vi "Read Rectangle.vi"(0 "GetPageSizeWithRotation":refnum<k24>, 7 "Pages dimensions [ ] IN":T1[](array[typedef]) {"Page Size" items=["Custom", "LETTER", "NOTE", "LEGAL", "TABLOID", "EXECUTIVE", "POSTCARD", "A0", "A1", "A2", "A3", "A4", "A5", "A6", "A7", "A8", "A9", "A10", "B0", "B1", "B2", "B3", "B4", "B5", "B6", "B7", "B8", "B9", "B10", "ARCH_E", "ARCH_D", "ARCH_C", "ARCH_B", "ARCH_A", "FLSA", "FLSE", "HALFLETTER", "_11X17", "ID_1", "ID_2", "ID_3", "LEDGER", "CROWN_QUARTO", "LARGE_CROWN_QUARTO", "DEMY_QUARTO", "ROYAL_QUARTO", "CROWN_OCTAVO", "LARGE_CROWN_OCTAVO", "DEMY_OCTAVO", "ROYAL_OCTAVO", "SMALL_PAPERBACK", "PENGUIN_SMALL_PAPERBACK", "PENGUIN_LARGE_PAPERBACK"]}, 11 "error in (no error)":errorcluster, 13 "Start at page":i32=1) -> (8 "Pages dimensions [ ] OUT":T1[](array[typedef]) {"Page Size" items=["Custom", "LETTER", "NOTE", "LEGAL", "TABLOID", "EXECUTIVE", "POSTCARD", "A0", "A1", "A2", "A3", "A4", "A5", "A6", "A7", "A8", "A9", "A10", "B0", "B1", "B2", "B3", "B4", "B5", "B6", "B7", "B8", "B9", "B10", "ARCH_E", "ARCH_D", "ARCH_C", "ARCH_B", "ARCH_A", "FLSA", "FLSE", "HALFLETTER", "_11X17", "ID_1", "ID_2", "ID_3", "LEDGER", "CROWN_QUARTO", "LARGE_CROWN_QUARTO", "DEMY_QUARTO", "ROYAL_QUARTO", "CROWN_OCTAVO", "LARGE_CROWN_OCTAVO", "DEMY_OCTAVO", "ROYAL_OCTAVO", "SMALL_PAPERBACK", "PENGUIN_SMALL_PAPERBACK", "PENGUIN_LARGE_PAPERBACK"]}, 15 "error out":errorcluster)   [LabVIEW 2019]
doc: "Developed by Jean-Marc Simard\nCopyright © 2012, Exaprom Inc.\nAll rights reserved.\nLicense: BSD\n\nWith iTextSharp 4.1.6 (http://itextsharp.sourceforge.net)\nunder Mozilla Public License Version 1.1\n(http://www.mozilla.org/MPL/MPL-1.1.html)"
uses:
  C:/Program Files/National Instruments/LabVIEW 2019/user.lib/Exaprom PDF/DLL/itextsharp.dll
  DLL/itextsharp.dll
  <userlib>/Exaprom PDF/Controls/Page Controls/Page dimensions.ctl
  <userlib>/Exaprom PDF/Controls/Page Controls/Page size.ctl
  <userlib>/Exaprom PDF/Controls/Page Controls/Page Orientation.ctl
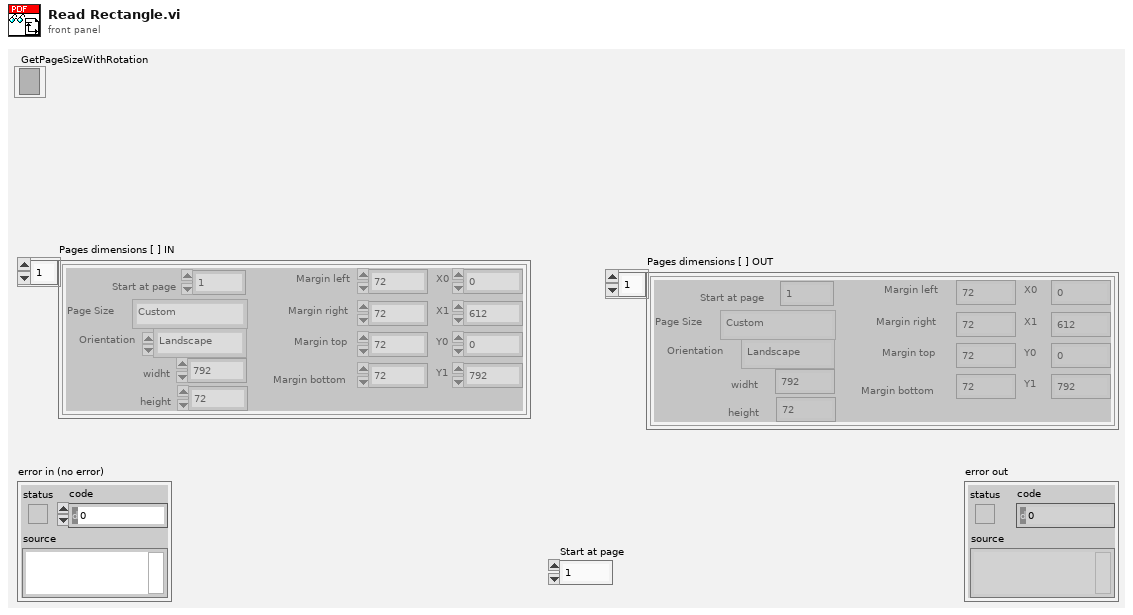
[diagram p1: front panel]
types:
  T1 = typedef "Page dimensions.ctl" = cluster{"Start at page":i32, "Page Size":T2, "Orientation":T3, "widht":sgl, "height":sgl, "Margin left":sgl, "Margin right":sgl, "Margin top":sgl, "Margin bottom":sgl, "X0":sgl, "X1":sgl, "Y0":sgl, "Y1":sgl}
  T2 = typedef "Page size.ctl" = i32
  T3 = typedef "Page Orientation.ctl" = enum16{"Portrait", "Landscape"}
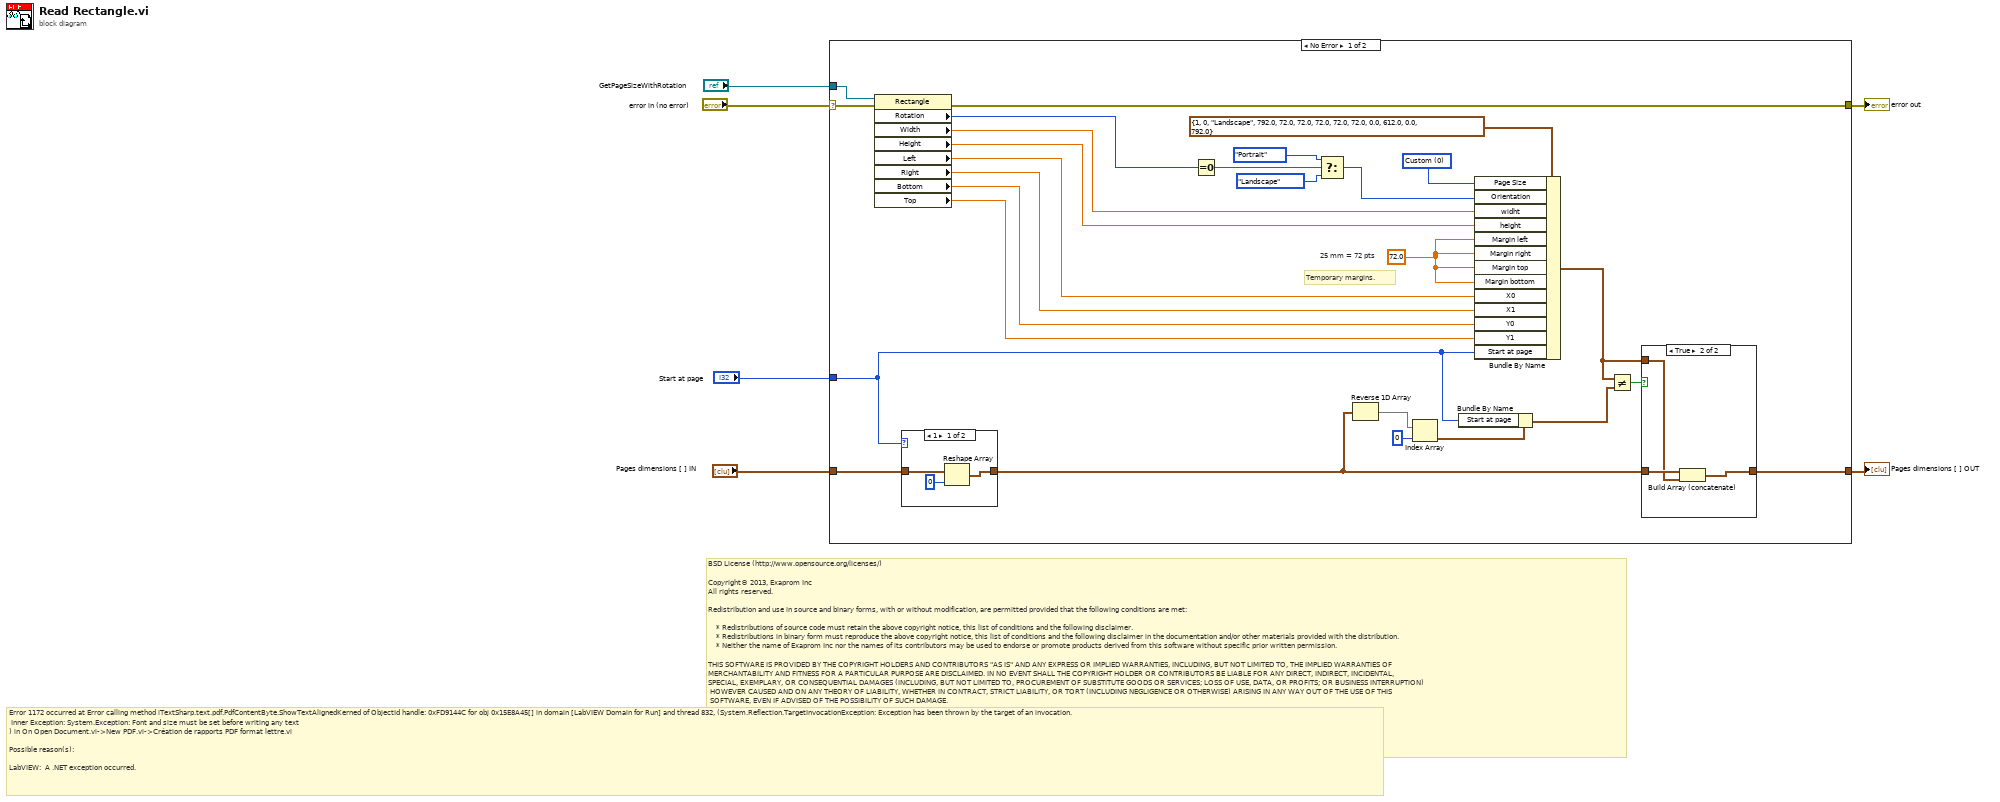
[diagram p0: block diagram]
diagram:
  # "Error 1172 occurred at Error calling method iTextSharp.text.pdf.PdfContentByte.ShowTextAlignedKerned of ObjectId handle: 0xFD9144C for obj 0x15E8A45[] in domain [LabVIEW Domain for Run] and thread 832, (System.Reflection.TargetInvocationException: Exception has been thrown by the target of an invocation.\n\tInner Exception: System.Exception: Font and size must be set before writing any text\n) in On Open Document.vi->New PDF.vi->Création de rapports PDF format lettre.vi\n\nPossible reason(s):\n\nLabVIEW:  A .NET exception occurred."
  # "BSD License (http://www.opensource.org/licenses/)\n\nCopyright© 2013, Exaprom Inc\nAll rights reserved.\n\nRedistribution and use in source and binary forms, with or without modification, are permitted provided that the following conditions are met:\n\n    * Redistributions of source code must retain the above copyright notice, this list of conditions and the following disclaimer.\n    * Redistributions in binary form must reproduce the above copyright notice, this list of conditions and the following disclaimer in the documentation and/or other materials provided with the distribution.\n    * Neither the name of Exaprom Inc nor the names of its contributors may be used to endorse or promote products derived from this software without specific prior written permission.\n\nTHIS SOFTWARE IS PROVIDED BY THE COPYRIGHT HOLDERS AND CONTRIBUTORS \"AS IS\" AND ANY EXPRESS OR IMPLIED WARRANTIES, INCLUDING, BUT NOT LIMITED TO, THE IMPLIED WARRANTIES OF \nMERCHANTABILITY AND FITNESS FOR A PARTICULAR PURPOSE ARE DISCLAIMED. IN NO EVENT SHALL THE COPYRIGHT HOLDER OR CONTRIBUTORS BE LIABLE FOR ANY DIRECT, INDIRECT, INCIDENTAL,\nSPECIAL, EXEMPLARY, OR CONSEQUENTIAL DAMAGES (INCLUDING, BUT NOT LIMITED TO, PROCUREMENT OF SUBSTITUTE GOODS OR SERVICES; LOSS OF USE, DATA, OR PROFITS; OR BUSINESS INTERRUPTION)\n HOWEVER CAUSED AND ON ANY THEORY OF LIABILITY, WHETHER IN CONTRACT, STRICT LIABILITY, OR TORT (INCLUDING NEGLIGENCE OR OTHERWISE) ARISING IN ANY WAY OUT OF THE USE OF THIS\n SOFTWARE, EVEN IF ADVISED OF THE POSSIBILITY OF SUCH DAMAGE."
  n1 = case shown="No Error" "error in (no error)" {
    selector: "error in (no error)" -> [w33 w42]
    tunnel: [w26 w42] -> w6
    tunnel: "GetPageSizeWithRotation" -> [w32 _]
    tunnel: "Start at page" -> [w7 _]
    tunnel: "Pages dimensions [ ] IN" -> [w10 _]
    tunnel: [w11 _] -> w1
    frame No Error {
      w21 = sgl 72.0  # 25 mm = 72 pts
      w24 = T2 0 items=["Custom", "LETTER", "NOTE", "LEGAL", "TABLOID", "EXECUTIVE", "POSTCARD", "A0", "A1", "A2", "A3", "A4", "A5", "A6", "A7", "A8", "A9", "A10", "B0", "B1", "B2", "B3", "B4", "B5", "B6", "B7", "B8", "B9", "B10", "ARCH_E", "ARCH_D", "ARCH_C", "ARCH_B", "ARCH_A", "FLSA", "FLSE", "HALFLETTER", "_11X17", "ID_1", "ID_2", "ID_3", "LEDGER", "CROWN_QUARTO", "LARGE_CROWN_QUARTO", "DEMY_QUARTO", "ROYAL_QUARTO", "CROWN_OCTAVO", "LARGE_CROWN_OCTAVO", "DEMY_OCTAVO", "ROYAL_OCTAVO", "SMALL_PAPERBACK", "PENGUIN_SMALL_PAPERBACK", "PENGUIN_LARGE_PAPERBACK"] ("Page Size")
      # "Temporary margins."
      n2 = property class="Rectangle"(reference=w32, error in=w33) -> (error out=w26:errorcluster, "Rotation"=w31:i32, "Width"=w23:sgl, "Height"=w22:sgl, "Left"=w20:sgl, "Right"=w19:sgl, "Bottom"=w18:sgl, "Top"=w17:sgl)  [unwired: 1 out]
      n3 = case shown="1" w7 {
        tunnel: w10 -> [w36 w37]
        tunnel: [w35 w37] -> w8
        frame 1 {
          n4 = Reshape Array(w36, 0 ("dimension size")) -> (w35:T1[])
        }
        frame 2.., Default {
        }
      }
      n5 = Equal To 0?(x=w31) -> (x = 0?=w30:bool)
      n6 = Select(t=Page_Orientation."Portrait" ("Orientation"), s=w30, f=Page_Orientation."Landscape" ("Orientation")) -> (s? t:f=w25:T3)
      n7 = Reverse 1D Array(array=w8) -> (reversed array=w16:T1[])
      n8 = Index Array(array=w16, index=0) -> (element=w14:T1)
      n9 = Bundle By Name(cluster=w14, "Start at page"=w7) -> (w13:T1)
      n10 = Bundle By Name(cluster=T1 {"Start at page"=1, "Page Size"=0, "Orientation"=enum."Landscape", "widht"=792.0, "height"=72.0, "Margin left"=72.0, "Margin right"=72.0, "Margin top"=72.0, "Margin bottom"=72.0, "X0"=0.0, "X1"=612.0, "Y0"=0.0, "Y1"=792.0} ("Page (points)"), "Page Size"=w24, "Orientation"=w25, "widht"=w23, "height"=w22, "Margin left"=w21, "Margin right"=w21, "Margin top"=w21, "Margin bottom"=w21, "X0"=w20, "X1"=w19, "Y0"=w18, "Y1"=w17, "Start at page"=w7) -> (w9:T1)
      n11 = Not Equal?(x=w9, y=w13) -> (x != y?=w12:bool)
      n12 = case shown="True" w12 {
        tunnel: [w38 w39] -> w11
        tunnel: w8 -> [w38 w41]
        tunnel: w9 -> [_ w40]
        frame False {
        }
        frame True {
          n13 = Build Array (concatenate)(w41, w40) -> (w39:T1[])
        }
      }
    }
    frame Error {
    }
  }
  "error out" <- w6
  "Pages dimensions [ ] OUT" <- w1
